vi "FPGA Init.vi"(8 "error in (no error)":errorcluster, 11 "Item Ref in":T1 format="%.0x") -> (0 "error out":errorcluster, 2 "FPGA Session Out":refnum<class "FPGA Interface Base.lvclass">, 3 "Item Ref Out":T1 format="%.0x")   [LabVIEW 2011, in "Sensor Simulation Custom Device.lvlib"]
uses:
  Sensor Simulation Custom Device.lvlib
  <vilib>/NI Veristand/Custom Device API/Custom Device Item Ref.ctl
  <userlib>/_FPGA Interface Advanced Tools/FPGA Interface Base/FPGA Interface Base.lvclass
  <userlib>/_FPGA Interface Advanced Tools/FPGA Interface Wrapper/TypeDefs/Open Attribute.ctl
  <vilib>/NI Veristand/Custom Device API/Get Item Property (Path).vi
  <vilib>/NI Veristand/Custom Device API/Get Item Property (Boolean).vi
  <vilib>/NI Veristand/Custom Device API/Get Item Property (String).vi
  Global.vi
  <vilib>/NI Veristand/Custom Device API/Custom Device API.lvlib
  <userlib>/_FPGA Interface Advanced Tools/FPGA Interface Wrapper/FPGA Interface Wrapper.lvlib
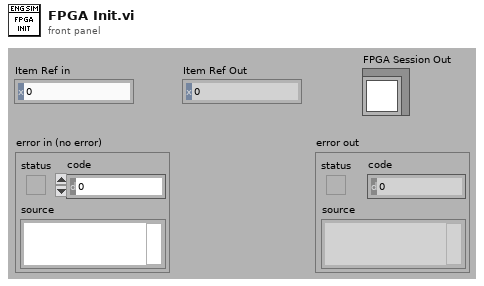
[diagram p1: front panel]
types:
  T1 = typedef "Custom Device API.lvlib/Custom Device Item Ref.ctl" = u64
  T2 = typedef "FPGA Interface Wrapper.lvlib/Open Attribute.ctl" = enum32{"Run (Default)", "No Run"}
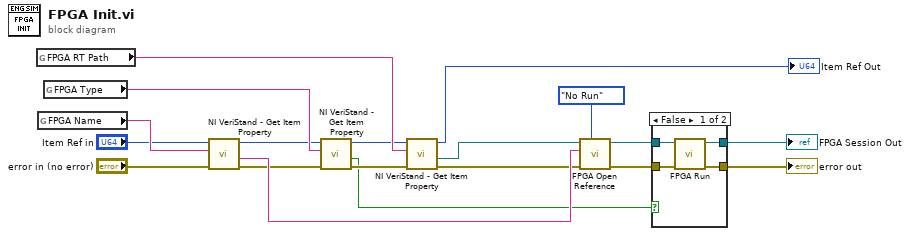
[diagram p0: block diagram]
diagram:
  n1 = global read "Global.vi" "FPGA RT Path"() -> (w19:string)
  n2 = global read "Global.vi" "FPGA Name"() -> (w18:string)
  n3 = global read "Global.vi" "FPGA Type"() -> (w15:string)
  n4 = call-poly <vilib>:"NI VeriStand - Get Item Property.vi"("error in (no error)"="error in (no error)", "Property Name"=w18, "Item Ref in"="Item Ref in") -> ("error out"=w8:errorcluster, "Value"=w11:string, "Item Ref out"=w7:T1)  [unwired: 5 in, 1 out]
  n5 = call-poly <vilib>:"NI VeriStand - Get Item Property.vi"("error in (no error)"=w8, "Property Name"=w15, "Item Ref in"=w7) -> ("error out"=w5:errorcluster, "Value"=w4:bool, "Item Ref out"=w6:T1)  [unwired: 5 in, 1 out]
  n6 = call-poly <vilib>:"NI VeriStand - Get Item Property.vi"("error in (no error)"=w5, "Property Name"=w19, "Item Ref in"=w6) -> ("error out"=w10:errorcluster, "Value"=w1:path, "Item Ref out"=→"Item Ref Out":T1)  [unwired: 5 in, 1 out]
  n7 = call <userlib>:"FPGA Open Reference.vi"("Run?"=Open_Attribute."No Run", "error in (no error)"=w10, "FPGA Resource"=w11, "Bitfile Path"=w1) -> ("error out"=w3:errorcluster, "FPGA Session"=w2:refnum<class "FPGA Interface Base.lvclass">)  [unwired: 6 in]
  n8 = case shown="False" w4 {
    tunnel: w2 -> [w23 w25]
    tunnel: w3 -> [w22 w24]
    tunnel: [w21 w24] -> w17
    tunnel: [w20 w25] -> w16
    frame False {
      n9 = call <userlib>:"FPGA Run.vi"("error in (no error)"=w22, "FPGA Session In"=w23) -> ("error out"=w21:errorcluster, "FPGA Session Out"=w20:refnum<class "FPGA Interface Base.lvclass">)  [unwired: 8 in]
    }
    frame True {
    }
  }
  "error out" <- w17
  "FPGA Session Out" <- w16
